vi "build refresh token URI.vi"(8 "error in (no error)":errorcluster, 11 "Oauth2.Google in":refnum<class "Oauth2.Google.lvclass">) -> (0 "error out":errorcluster, 2 "Refresh Token Request URI":string, 3 "Oauth2.Google":refnum<class "Oauth2.Google.lvclass">)   [LabVIEW 2017, in "Oauth2.Google.lvclass"]
uses:
  Oauth2.Google.lvclass
  D:/GitHub/Oauth2/source/Oauth2/Oauth2.lvclass
  OAuthToken/OAuth2 Token Element -- enum.ctl
  Oauth2/Oauth2.lvclass/Oauth2.ctl
  OAuthToken/OAuthAccessToken.lvclass
  <vilib>/LabVIEW Open Source Project/OpenURI/uri/URI.lvclass
  Oauth2/Oauth2.lvclass
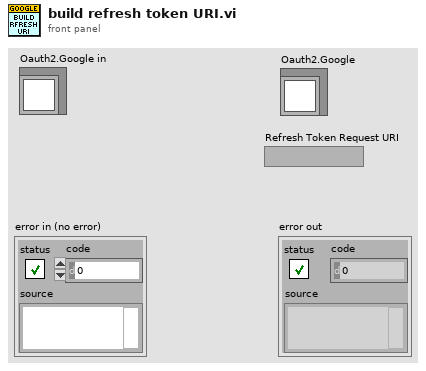
[diagram p1: front panel]
types:
  T1 = typedef "OAuthAccessToken.lvclass/OAuth2 Token Element -- enum.ctl" = enum16{"client_id", "client_secret", "response_type", "scope", "redirect_uri", "error", "error_description", "error_uri", "grant_type", "code", "access_token", "token_type", "expires_in", "username", "password", "refresh_token", "code_challenge", "code_challenge_method", "reverse_proxy_uri", "endpoint element", "prompt", "access_type", "id_token"}
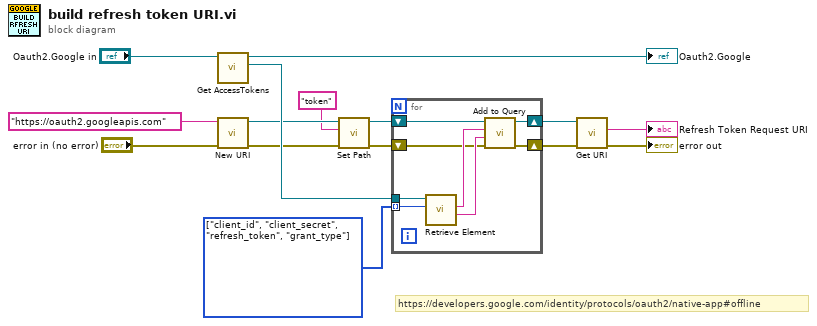
[diagram p0: block diagram]
diagram:
  w15 = T1[] [enum."client_id", enum."client_secret", enum."refresh_token", enum."grant_type"] items=["client_id", "client_secret", "response_type", "scope", "redirect_uri", "error", "error_description", "error_uri", "grant_type", "code", "access_token", "token_type", "expires_in", "username", "password", "refresh_token", "code_challenge", "code_challenge_method", "reverse_proxy_uri", "endpoint element", "prompt", "access_type", "id_token"]
  # "https://developers.google.com/identity/protocols/oauth2/native-app#offline"
  n1 = call "Get AccessTokens.vi"("Oauth2 in"="Oauth2.Google in") -> ("OAuthAccessToken"=w9:refnum<class "OAuthAccessToken.lvclass">, "Oauth2 out"=→"Oauth2.Google":refnum<class "Oauth2.Google.lvclass">)  [unwired: 8 in, 1 out]
  n2 = call <vilib>:"New URI.vi"("error in (no error)"="error in (no error)", "URI"="https://oauth2.googleapis.com") -> ("error out"=w8:errorcluster, "URI"=w6:refnum<class "URI.lvclass">)  [unwired: 8 in]
  n3 = call <vilib>:"Set Path.vi"("error in (no error)"=w8, "path"="token", "URI in"=w6) -> ("error out"=w11:errorcluster, "URI out"=w14:refnum<class "URI.lvclass">)  [unwired: 7 in]
  n4 = for {
    tunnel: w9 -> [w23]
    tunnel: w15 -> [w22] mode=indexing
    shift-right: [w20] -> w13
    shift-left: w14 -> [w21]
    shift-right: [w16] -> w12
    shift-left: w11 -> [w17]
    n5 = call "Retrieve Element.vi"("Token element"=w22, "OAuthAccessToken in"=w23) -> ("Value"=w18:string, "Key"=w19:string)  [unwired: 5 in, 3 out]
    n6 = call <vilib>:"Add to Query.vi"("error in (no error)"=w17, "value"=w18, "key"=w19, "URI in"=w21) -> ("error out"=w16:errorcluster, "URI out"=w20:refnum<class "URI.lvclass">)  [unwired: 6 in]
  }
  n7 = call <vilib>:"Get URI.vi"("error in (no error)"=w12, "URI in"=w13) -> ("error out"=→"error out":errorcluster, "URI String"=→"Refresh Token Request URI":string)  [unwired: 7 in, 1 out]
